vi "APS start task.vi"(8 "error in (no error)":errorcluster caption="错误输入（无错误）", 9 "CtrlCmd":i32, 10 "TaskNum":i32, 11 "Board_ID":i32) -> (0 "error out":errorcluster caption="错误输出", 3 "function return":i32)   [LabVIEW 2011, in "APS168.lvlib"]
doc: "I32 FNTYPE APS_start_task( I32 Board_ID, I32 TaskNum, I32 CtrlCmd );"
uses:
  APS168.lvlib
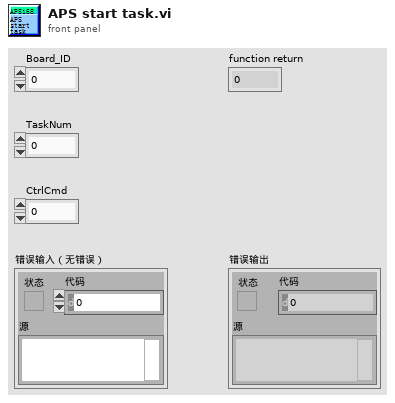
[diagram p1: front panel]
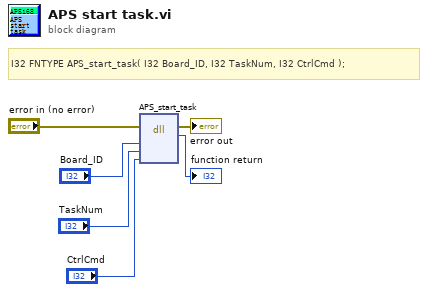
[diagram p0: block diagram]
diagram:
  # "I32 FNTYPE APS_start_task( I32 Board_ID, I32 TaskNum, I32 CtrlCmd );"
  n1 = dll-call lib="PTH1Labs E软件ADLINK 204CAPS_1_7_1_LIB line 连续运动204APS168.*" fn="APS_start_task"(error in="error in (no error)", "Board_ID"="Board_ID", "TaskNum"="TaskNum", "CtrlCmd"="CtrlCmd") -> (error out=→"error out":errorcluster, →"function return":i32)  [unwired: 5 in, 1 out]
